vi "Station3_Data_Log.vi"(0 "Cluster":T2, 3 "error in (no error)":errorcluster) -> (10 "error out":errorcluster)   [LabVIEW 2017]
uses:
  <vilib>/addons/database/Connection.llb/Conn ObjectReference.ctl
  <vilib>/addons/database/NI_Database_API.lvlib
panel:
  out "PART 1":string
  out "PART 2":string
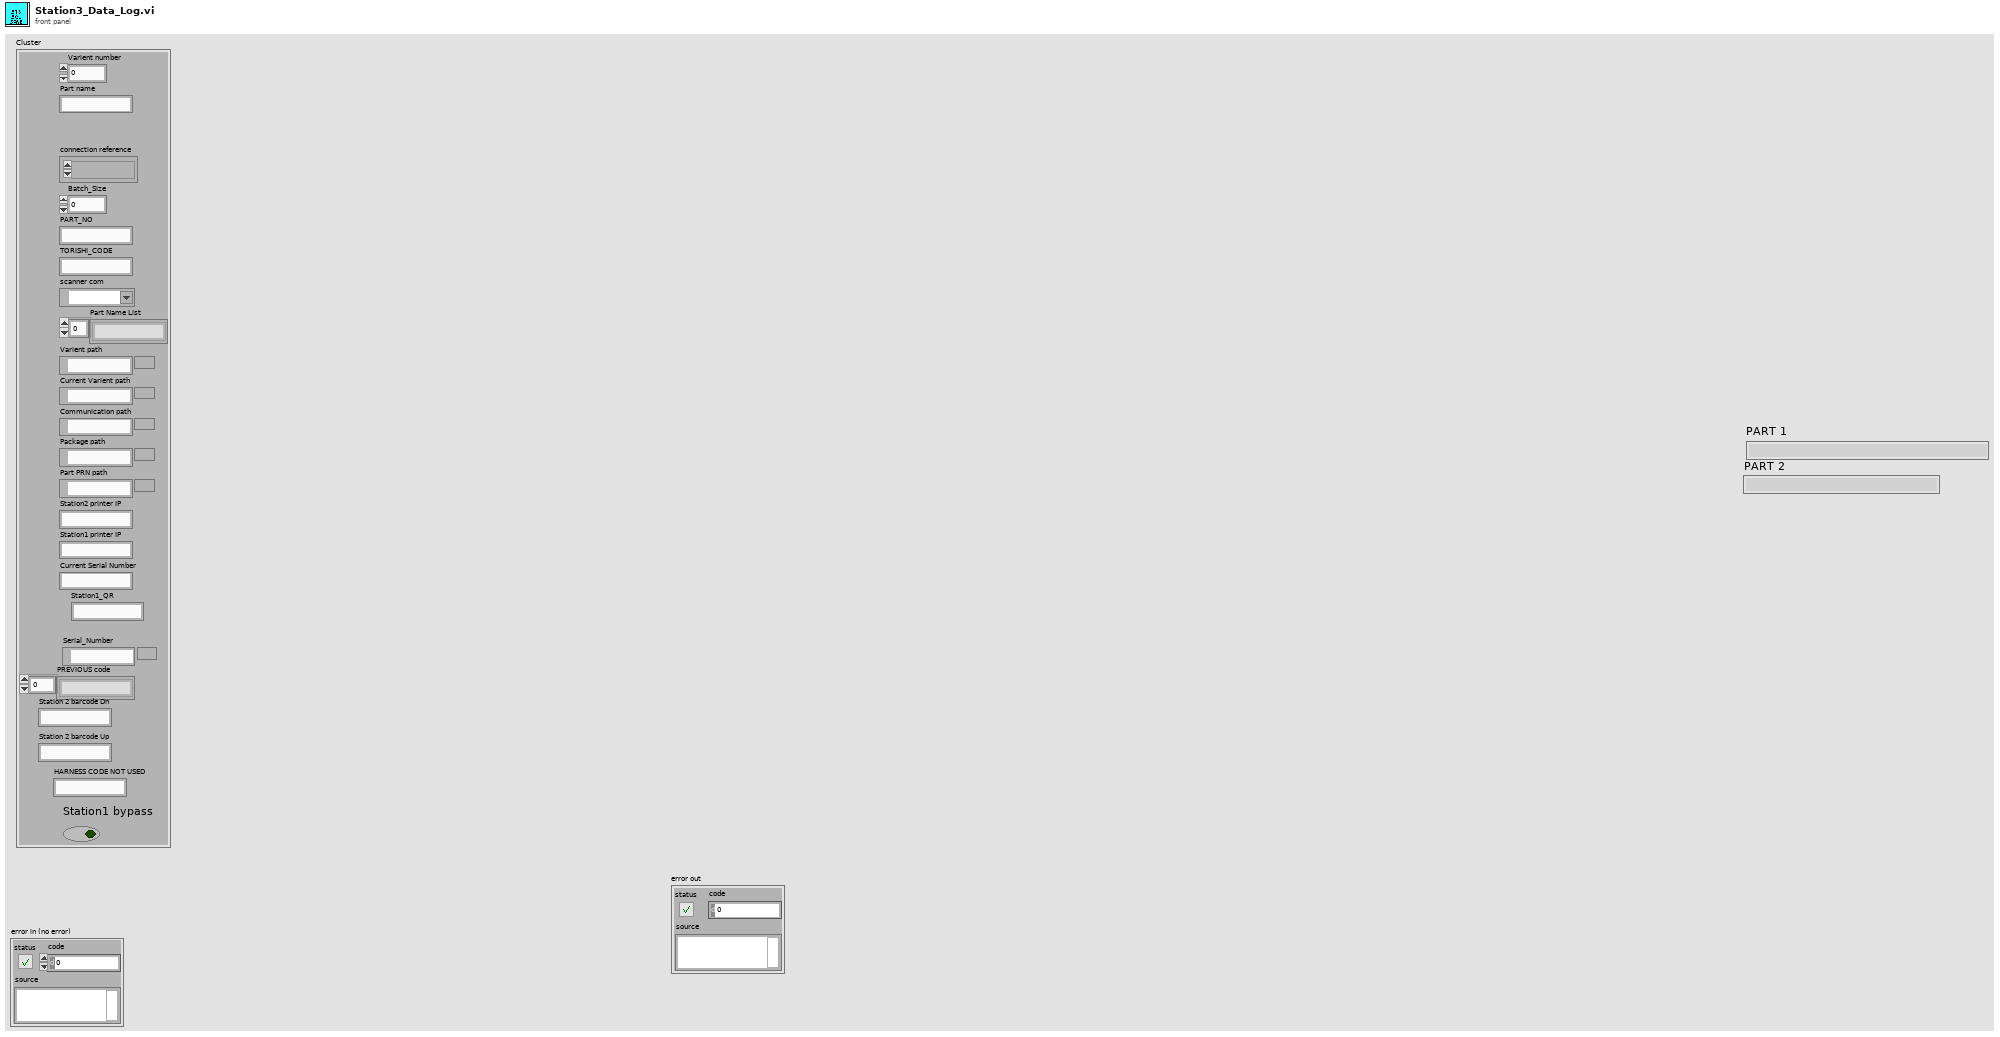
[diagram p1: front panel]
types:
  T1 = typedef "NI_Database_API.lvlib/Conn ObjectReference.ctl" = refnum<k1>
  T2 = cluster{"Varient number":u16, "Part name":string, "connection reference":T1, "Batch_Size":u16, "PART_NO":string, "TORISHI_CODE":string, "scanner com":refnum<visa-resource-name>, "Part Name List":string[], "Varient path":path, "Current Varient path":path, "Communication path":path, "Package path":path, "Part PRN path":path, "Station2 printer IP":string, "Station1 printer IP":string, "Current Serial Number":string, "Station1_QR":string, "Serial_Number":path, "PREVIOUS code":string[], "Station 2 barcode Dn":string, "Station 2 barcode Up":string, "HARNESS CODE NOT USED":string, "Station1 bypass":bool}
  T3 = cluster{string, "Station 2 barcode Up":string, "Station 2 barcode Dn":string}
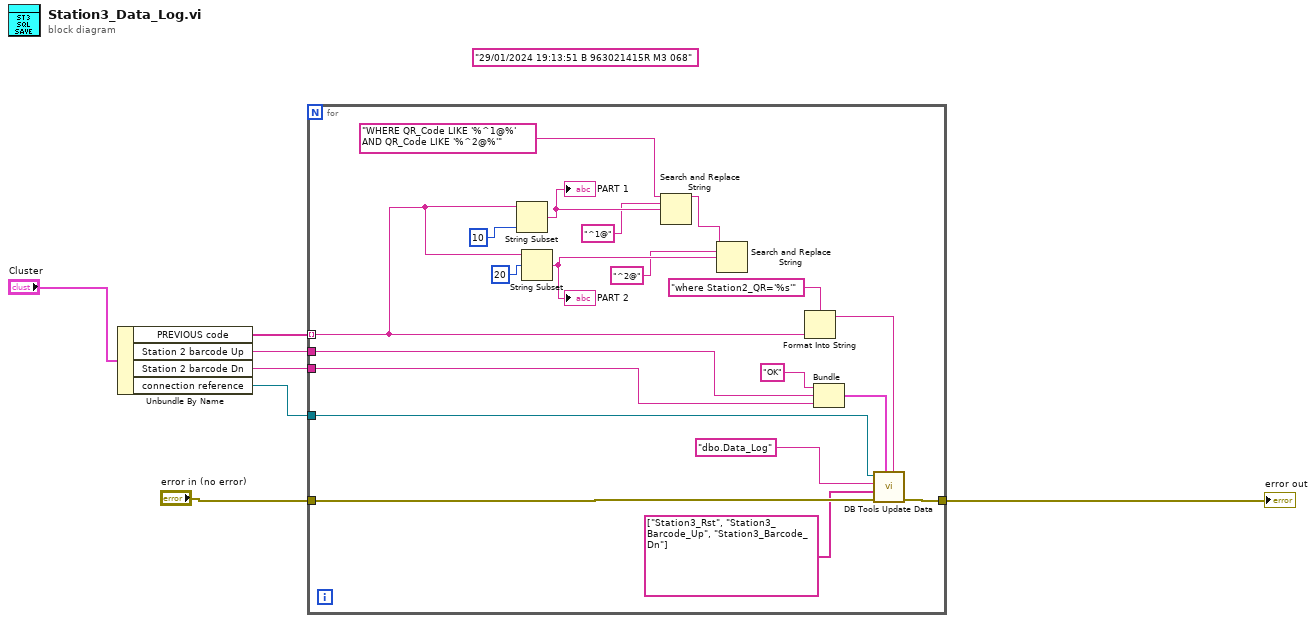
[diagram p0: block diagram]
diagram:
  (unwired) "29/01/2024 19:13:51 B 963021415R M3 068"
  n1 = Unbundle By Name("Cluster") -> ("PREVIOUS code"=w5:string[], "Station 2 barcode Up"=w4:string, "Station 2 barcode Dn"=w3:string, "connection reference"=w2:T1)
  n2 = for {
    tunnel: [w26] -> w7
    tunnel: w2 -> [w25]
    tunnel: "error in (no error)" -> [w22]
    tunnel: w5 -> [w10] mode=indexing
    tunnel: w4 -> [w21]
    tunnel: w3 -> [w20]
    n3 = String Subset(string=w10, length (rest)=10 ("offset (0)")) -> (substring=w17:string)  [unwired: 1 in]
    "PART 1" <- w17
    n4 = String Subset(string=w10, offset (0)=20) -> (substring=w18:string)  [unwired: 1 in]
    "PART 2" <- w18
    n5 = Search and Replace String(input string="WHERE QR_Code LIKE '%^1@%' AND QR_Code LIKE '%^2@%'" ("format string"), search string="^1@", replace string=w17) -> (result string=w16:string)  [unwired: 5 in, 3 out]
    n6 = Search and Replace String(input string=w16, search string="^2@", replace string=w18) -> ()  [unwired: 5 in, 4 out]
    n7 = Format Into String(format string="where Station2_QR='%s'", w10) -> (resulting string=w8:string)  [unwired: 2 in, 1 out]
    n8 = Bundle("OK", "Station 2 barcode Up"=w21, "Station 2 barcode Dn"=w20) -> (w23:T3)  [unwired: 1 in]
    n9 = call <vilib>:"DB Tools Update Data.vi"("condition"=w8, "data"=w23, "error in (no error)"=w22, "columns"=string[] ["Station3_Rst", "Station3_Barcode_Up", "Station3_Barcode_Dn"] ("columns 2"), "table"="dbo.Data_Log", "connection reference"=w25) -> ("error out"=w26:errorcluster)  [unwired: 4 in, 1 out]
  }
  "error out" <- w7
